vi "Pre Launch Init.vi"(11 "Nested in":refnum<class "CheckPasswordUI.lvclass">) -> (0 "error out":errorcluster, 3 "Nested out":refnum<class "CheckPasswordUI.lvclass">)   [LabVIEW 2021, in "CheckPasswordUI.lvclass"]
doc: "(<B>Filename</B>: Actor Framework.lvlib:Actor.lvclass:Pre Launch Init.vi)\n\nDefines behavior that occurs after the Launch Nested Actor method is invoked but before the actor's Actor Core method begins running.\n\nBy default, this method does nothing. A descendant class may override it to define behavior."
uses:
  CheckPasswordUI.lvclass
  CheckPasswordUI.lvclass/CheckPasswordUI.ctl
  <userlib>/John_Lib/AbstractActorTemplate/AbstractActorTemplate/UIActorTop.lvclass
  <userlib>/John_Lib/Queue_Self/Queue_Self.lvlib
  DVR.ctl
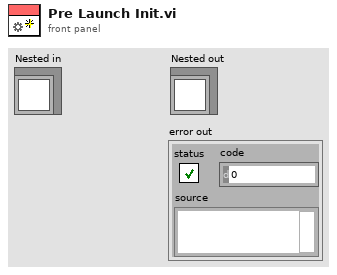
[diagram p1: front panel]
types:
  T1 = typedef "CheckPasswordUI.lvclass/DVR.ctl" = cluster{"Caller ActorQName":string}
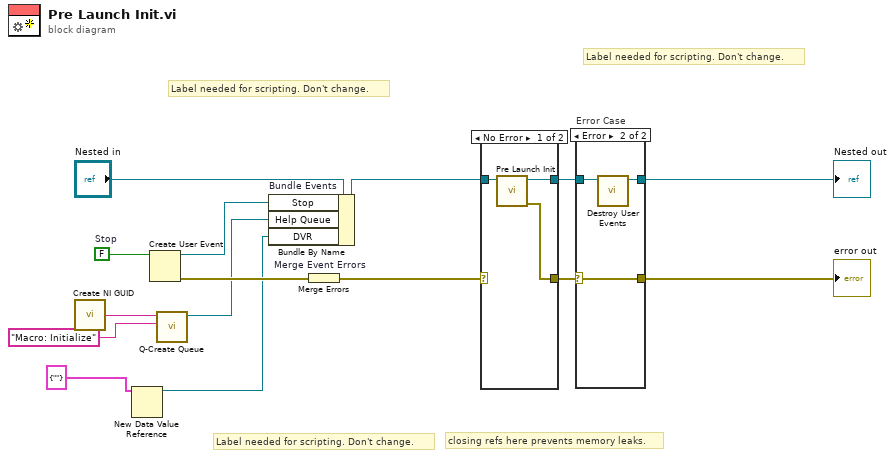
[diagram p0: block diagram]
diagram:
  w14 = FALSE  # Stop
  # "Label needed for scripting. Don't change."
  # "Label needed for scripting. Don't change."
  # "Label needed for scripting. Don't change."
  # "closing refs here prevents memory leaks."
  n1 = call <vilib>:"Create NI GUID.vi"() -> ("NI GUID"=w4:string)
  n2 = New Data Value Reference(data value=T1 {"Caller ActorQName"=""} ("DVR")) -> (data value reference=w1:refnum<data-value>)  [unwired: 1 in, 1 out]
  n3 = Create User Event(user event datatype=w14) -> (user event=w11:refnum<user-event>, error out=w13:errorcluster)  [unwired: 1 in]
  n4 = call <userlib>:"Q-Create Queue.vi"("CMD"="Macro: Initialize" ("initial message names"), "message queue name"=w4) -> ("queue out"=w3:refnum<queue>)  [unwired: 8 in, 1 out]
  n5 = Bundle By Name "Bundle Events"(cluster="Nested in", "Stop"=w11, "Help Queue"=w3, "DVR"=w1) -> (w8:refnum<class "CheckPasswordUI.lvclass">)
  n6 = Merge Errors "Merge Event Errors"(w13) -> (w7:errorcluster)
  n7 = case shown="No Error" w7 {
    selector: w7 -> [_ w20]
    tunnel: [w18 w19] -> w9
    tunnel: w8 -> [w17 w19]
    tunnel: [w16 w20] -> w6
    frame No Error {
      n8 = call-parent "Pre Launch Init.vi"("Actor in"=w17) -> ("error out"=w16:errorcluster, "Actor out"=w18:refnum<class "CheckPasswordUI.lvclass">)  [unwired: 9 in]
    }
    frame Error {
    }
  }
  n9 = case "Error Case" shown="Error" w6 {
    selector: w6 -> [w21 w25]
    tunnel: w9 -> [w22 w24]
    tunnel: [w22 w23] -> w12
    tunnel: [w21 w25] -> w10
    frame No Error {
    }
    frame Error {
      n10 = call "Destroy User Events.vi"("UI Template in"=w24) -> ("UI Template out"=w23:refnum<class "CheckPasswordUI.lvclass">)  [unwired: 10 in]
    }
  }
  "error out" <- w10
  "Nested out" <- w12
